vi "Program Stop.vi"(0 "GUI error":errorcluster, 4 "user interface":refnum<queue>, 5 "user event":refnum<user-event>, 6 "operation error":errorcluster, 7 "Event Registration Refnum":refnum<event-registration>, 8 "FP control error":errorcluster, 11 "user events":refnum<queue>) -> ()   [LabVIEW 2011]
uses:
  Controls/User Event Control.ctl
  Controls/User Event Action.ctl
  Controls/User Interface Control.ctl
  Controls/User Interface Action.ctl
  Error Handling/Error Module Action.ctl
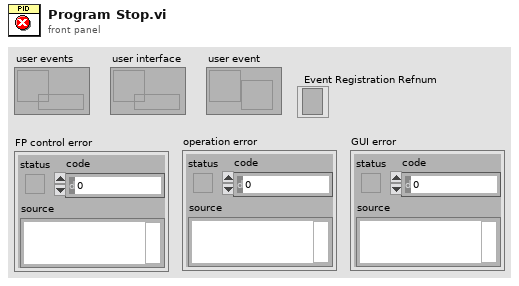
[diagram p1: front panel]
types:
  T1 = typedef "Error Module Action.ctl" = enum16{"Initialize", "Handle Errors", "Report Errors"}
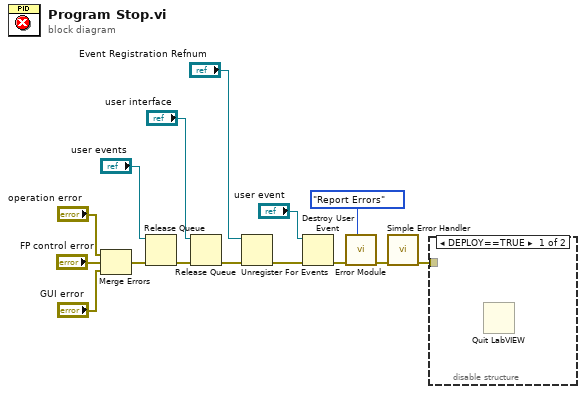
[diagram p0: block diagram]
diagram:
  n1 = Merge Errors("operation error", "FP control error", "GUI error") -> (w12:errorcluster)
  n2 = Release Queue(queue="user events", error in (no error)=w12) -> (error out=w13:errorcluster)  [unwired: 1 in, 2 out]
  n3 = Release Queue(queue="user interface", error in (no error)=w13) -> (error out=w3:errorcluster)  [unwired: 1 in, 2 out]
  n4 = Unregister For Events(event registration refnum="Event Registration Refnum", error in=w3) -> (error out=w14:errorcluster)
  n5 = Destroy User Event(user event="user event", error in=w14) -> (error out=w7:errorcluster)
  n6 = call "Error Module.vi"("Command (Handle Errors"=Error_Module_Action."Report Errors", "error in"=w7) -> ("error out"=w6:errorcluster)  [unwired: 8 in, 1 out]
  n7 = call <vilib>:"Simple Error Handler.vi"("error in (no error)"=w6) -> ("error out"=w15:errorcluster)  [unwired: 4 in, 4 out]
  n8 = disable-structure shown="DEPLOY==TRUE" {
    disable-tunnel: w15 -> [_ _]
    frame condition #0 {
      n9 = Quit LabVIEW() -> ()  [unwired: 1 in]
    }
    frame condition #1 (active) {
    }
  }
